vi "System_Configuration_Get.vi"(3 "error in (no error)":errorcluster, 4 "Device Selection":T1, 5 "Devices":T2) -> (0 "error out":errorcluster, 2 "Config":T3 {"Compute Config"."Post-Trigger Time" format="%.3f ms"; "Compute Config"."Pre-Trigger Time" format="%.3f ms"; "Compute Config"."Trigger Frequency" items=["Single", "Continuous"]; "Compute Config"."Trigger Type" items=["GPS Time", "Anomaly Detection"]; "SDR Config"."WRx 2\nGain Attenuation" min=0 max=27 step=1 scale=0.0..27.0; "SDR Config"."WRx 2\nRSSI Threshold" format="%.2f dBm"; "SDR Config"."WRx 2\nGain Mode" items=["Automatic", "Fixed"]; "SDR Config"."WRx 2\nBandwidth Mode" items=["500 MHz"]; "SDR Config"."WRx 2\nIF Frequency" items=["1200 MHz", "1400 MHz", "3000 MHZ"]; "SDR Config"."WRx 1\nGain Attenuation" min=0 max=27 step=1 scale=0.0..27.0; "SDR Config"."WRx 1\nRSSI Threshold" format="%.2f dBm"; "SDR Config"."WRx 1\nGain Mode" items=["Automatic", "Fixed"]; "SDR Config"."WRx 1\nBandwidth Mode" items=["500 MHz"]; "SDR Config"."WRx 1\nIF Frequency" items=["1200 MHz", "1400 MHz", "3000 MHZ"]})   [LabVIEW 2024]
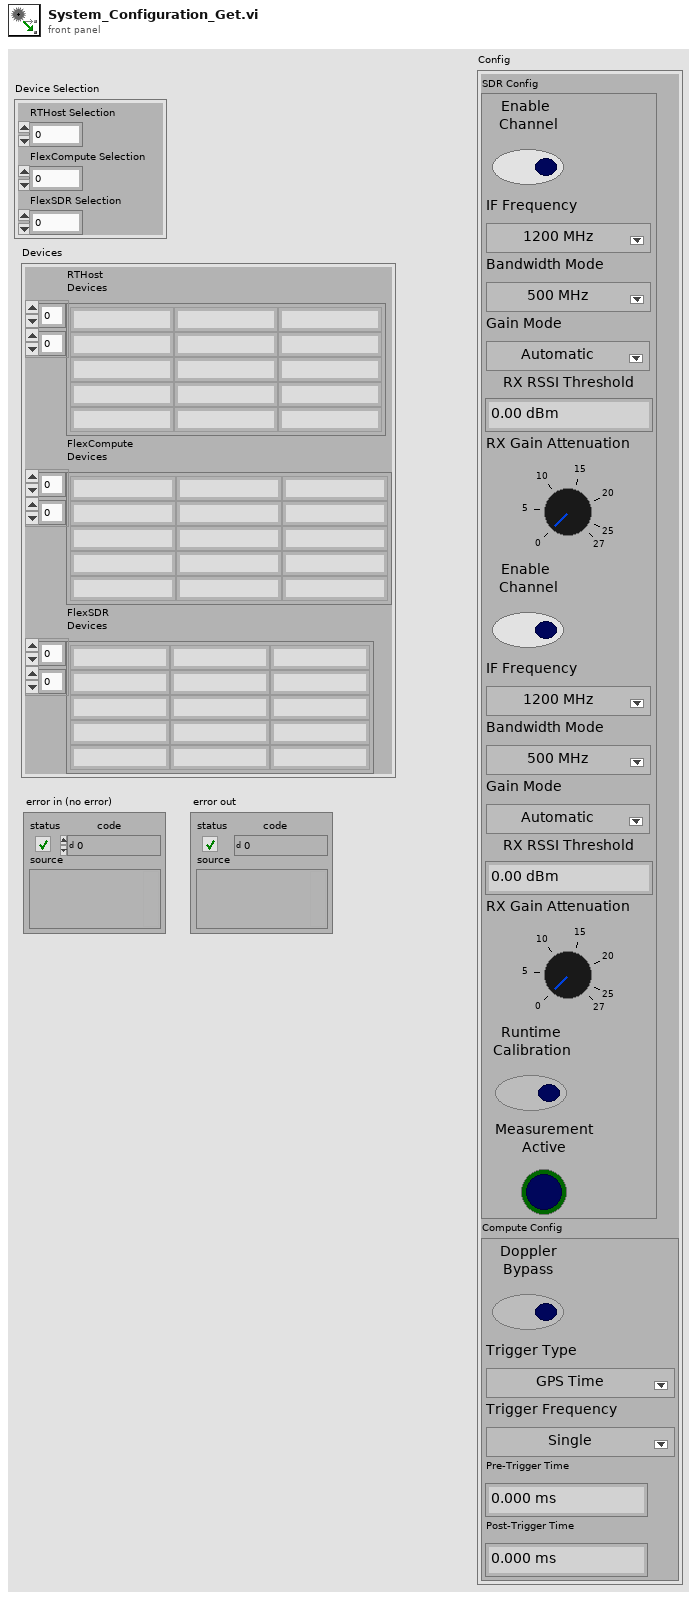
[diagram p1: front panel]
types:
  T1 = cluster{"RTHost Selection":u16, "FlexCompute Selection":u16, "FlexSDR Selection":u16}
  T2 = cluster{"RTHost\nDevices":string[][], "FlexCompute\nDevices":string[][], "FlexSDR\nDevices":string[][]}
  T3 = cluster{"SDR Config":cluster{"WRx 1\nEnable Channel":bool, "WRx 1\nIF Frequency":u16, "WRx 1\nBandwidth Mode":u16, "WRx 1\nGain Mode":u16, "WRx 1\nRSSI Threshold":dbl, "WRx 1\nGain Attenuation":i64, "WRx 2\nEnable Channel":bool, "WRx 2\nIF Frequency":u16, "WRx 2\nBandwidth Mode":u16, "WRx 2\nGain Mode":u16, "WRx 2\nRSSI Threshold":dbl, "WRx 2\nGain Attenuation":i64, "Runtime\nCalibration":bool, "Measurement\nActive":bool}, "Compute Config":cluster{"Doppler\nBypass":bool, "Trigger Type":u16, "Trigger Frequency":u16, "Pre-Trigger Time":dbl, "Post-Trigger Time":dbl}}
  T4 = cluster{"Doppler\nBypass":bool, "Trigger Type":u16, "Trigger Frequency":u16, "Pre-Trigger Time":dbl, "Post-Trigger Time":dbl}
  T5 = cluster{"WRx 1\nEnable Channel":bool, "WRx 1\nIF Frequency":u16, "WRx 1\nBandwidth Mode":u16, "WRx 1\nGain Mode":u16, "WRx 1\nRSSI Threshold":dbl, "WRx 1\nGain Attenuation":i64, "WRx 2\nEnable Channel":bool, "WRx 2\nIF Frequency":u16, "WRx 2\nBandwidth Mode":u16, "WRx 2\nGain Mode":u16, "WRx 2\nRSSI Threshold":dbl, "WRx 2\nGain Attenuation":i64, "Runtime\nCalibration":bool, "Measurement\nActive":bool}
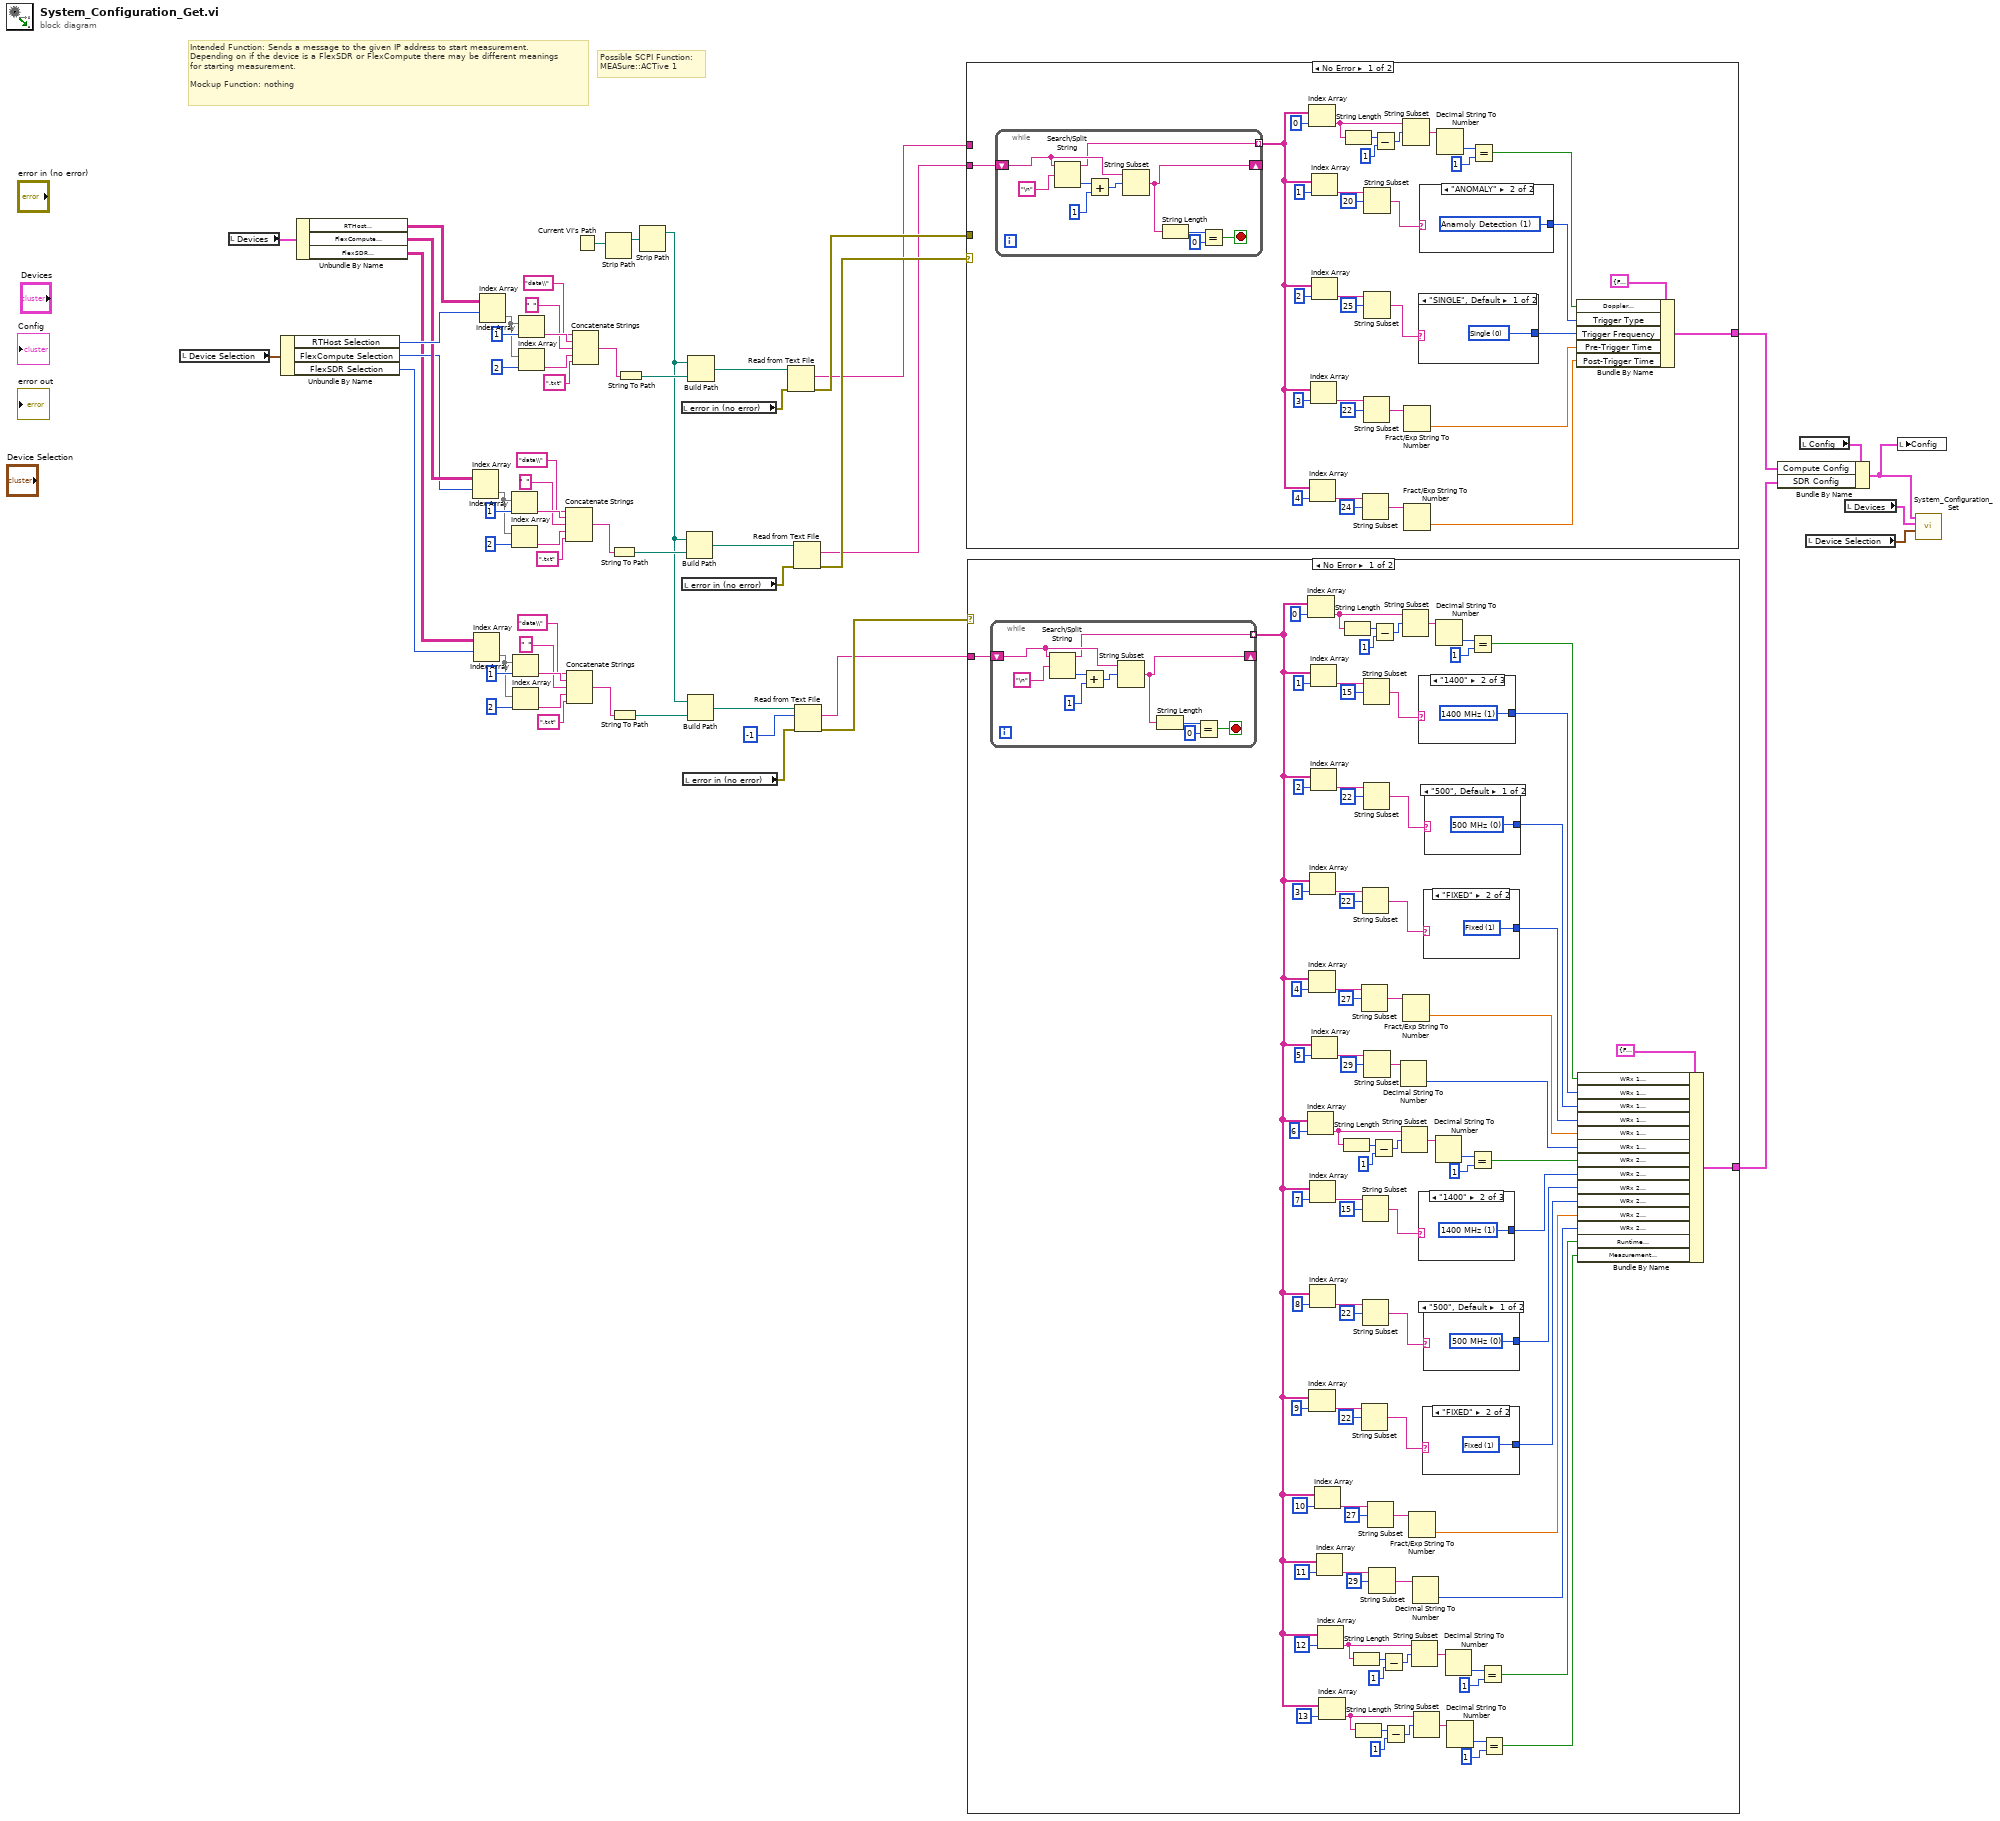
[diagram p0: block diagram]
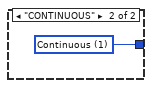
[diagram p2: hidden frame]
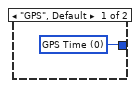
[diagram p3: hidden frame]
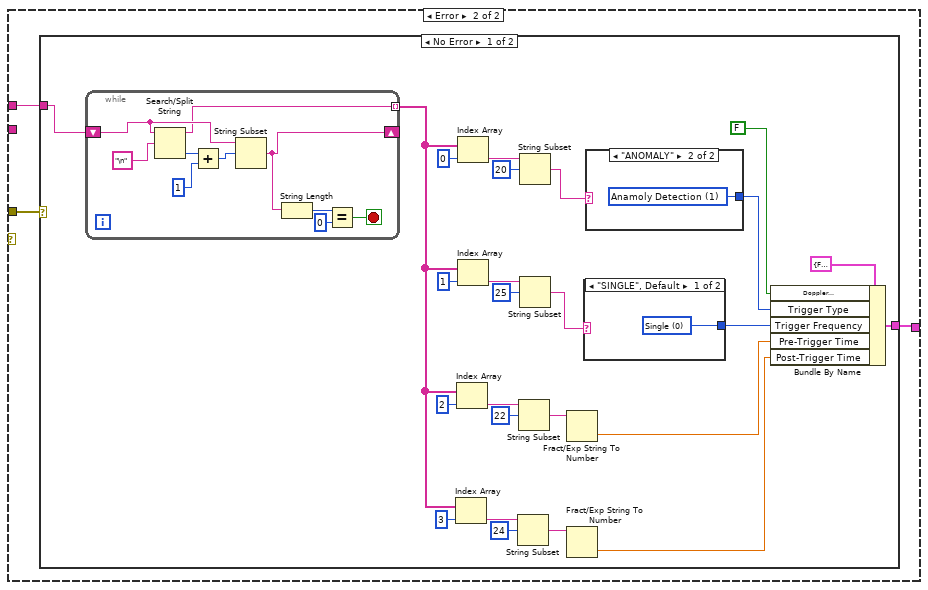
[diagram p4: hidden frame]
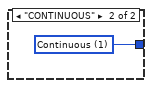
[diagram p5: hidden frame]
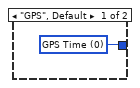
[diagram p6: hidden frame]
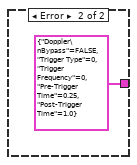
[diagram p7: hidden frame]
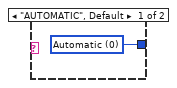
[diagram p8: hidden frame]
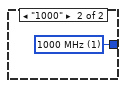
[diagram p9: hidden frame]
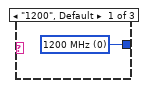
[diagram p10: hidden frame]
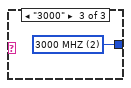
[diagram p11: hidden frame]
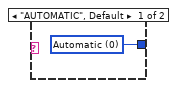
[diagram p12: hidden frame]
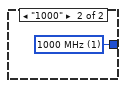
[diagram p13: hidden frame]
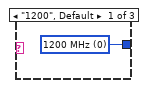
[diagram p14: hidden frame]
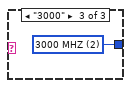
[diagram p15: hidden frame]
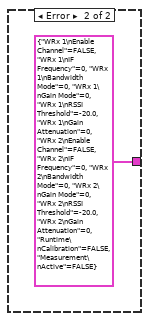
[diagram p16: hidden frame]
diagram:
  # "Possible SCPI Function:\nMEASure::ACTive 1"
  # "Intended Function: Sends a message to the given IP address to start measurement.\nDepending on if the device is a FlexSDR or FlexCompute there may be different meanings\nfor starting measurement.\n\nMockup Function: nothing"
  n1 = local read "Device Selection"() -> (w45:T1)
  n2 = local read "Devices"() -> (w49:T2)
  n3 = Unbundle By Name(w45) -> ("RTHost Selection"=w43:u16, "FlexCompute Selection"=w17:u16, "FlexSDR Selection"=w15:u16)
  n4 = Unbundle By Name(w49) -> ("RTHost\nDevices"=w44:string[][], "FlexCompute\nDevices"=w18:string[][], "FlexSDR\nDevices"=w16:string[][])
  n5 = Index Array(array=w18, index (row)=w17) -> (element=w41:string[])  [unwired: 1 in]
  n6 = Index Array(array=w16, index (row)=w15) -> (element=w29:string[])  [unwired: 1 in]
  n7 = Index Array(array=w44, index (row)=w43) -> (element=w58:string[])  [unwired: 1 in]
  n8 = Index Array(array=w41, index=1) -> (element=w39:string)
  n9 = Index Array(array=w41, index=2) -> (element=w38:string)
  n10 = Index Array(array=w29, index=1) -> (element=w27:string)
  n11 = Index Array(array=w29, index=2) -> (element=w26:string)
  n12 = Index Array(array=w58, index=1) -> (element=w56:string)
  n13 = Index Array(array=w58, index=2) -> (element=w55:string)
  n14 = Concatenate Strings("data\\" ("string"), w39, " " ("element"), w38, ".txt" ("string")) -> (w34:string)
  n15 = Concatenate Strings("data\\" ("string"), w27, " " ("element"), w26, ".txt" ("string")) -> (w22:string)
  n16 = Concatenate Strings("data\\" ("string"), w56, " " ("element"), w55, ".txt" ("string")) -> (w51:string)
  n17 = Current VI's Path() -> (path=w60:path)
  n18 = Strip Path(path=w60) -> (stripped path=w46:path)  [unwired: 1 out]
  n19 = String To Path(string=w34) -> (path=w33:path)
  n20 = String To Path(string=w22) -> (path=w21:path)
  n21 = String To Path(string=w51) -> (path=w50:path)
  n22 = Strip Path(path=w46) -> (stripped path=w19:path)  [unwired: 1 out]
  n23 = local read "error in (no error)"() -> (w48:errorcluster)
  n24 = local read "error in (no error)"() -> (w32:errorcluster)
  n25 = local read "error in (no error)"() -> (w20:errorcluster)
  n26 = Build Path(base path=w19, name or relative path=w33) -> (appended path=w31:path)
  n27 = Build Path(base path=w19, name or relative path=w21) -> (appended path=w11:path)
  n28 = Build Path(base path=w19, name or relative path=w50) -> (appended path=w47:path)
  n29 = Read from Text File(file (use dialog)=w47, error in=w48) -> (text=w7:string, error out=w14:errorcluster)  [unwired: 2 in, 2 out]
  n30 = Read from Text File(file (use dialog)=w31, error in=w32) -> (text=w8:string, error out=w13:errorcluster)  [unwired: 2 in, 2 out]
  n31 = Read from Text File(file (use dialog)=w11, count=-1, error in=w20) -> (text=w10:string, error out=w12:errorcluster)  [unwired: 1 in, 2 out]
  n32 = case shown="No Error" w13 {
    tunnel: w8 -> [w69 _]
    tunnel: w7 -> [_ w108]
    tunnel: w14 -> [_ w110]
    tunnel: [w61 w109] -> w5
    frame No Error {
      n33 = while {
        shift-right: [w99] -> _
        shift-left: w69 -> [w106]
        tunnel: [w98] -> w70 mode=indexing
        stop <- w100 stop-if-true
        n34 = Search/Split String(string=w106, search string/char (-)="\n") -> (substring before match=w98:string, offset of match=w105:i32)  [unwired: 1 in, 1 out]
        n35 = Add(x=w105, y=1) -> (x+y=w103:i32)
        n36 = String Subset(string=w106, offset (0)=w103) -> (substring=w99:string)  [unwired: 1 in]
        n37 = String Length(string=w99) -> (length=w102:i32)
        n38 = Equal?(x=w102, y=0) -> (x = y?=w100:bool)
      }
      n39 = Index Array(array=w70, index=0) -> (element=w90:string)
      n40 = Index Array(array=w70, index=4) -> (element=w73:string)
      n41 = Index Array(array=w70, index=3) -> (element=w76:string)
      n42 = Index Array(array=w70, index=1) -> (element=w84:string)
      n43 = Index Array(array=w70, index=2) -> (element=w80:string)
      n44 = String Length(string=w90) -> (length=w92:i32)
      n45 = String Subset(string=w73, offset (0)=24) -> (substring=w71:string)  [unwired: 1 in]
      n46 = String Subset(string=w76, offset (0)=22) -> (substring=w68:string)  [unwired: 1 in]
      n47 = String Subset(string=w84, offset (0)=20) -> (substring=w82:string)  [unwired: 1 in]
      n48 = String Subset(string=w80, offset (0)=25) -> (substring=w78:string)  [unwired: 1 in]
      n49 = Subtract(x=w92, y=1) -> (x-y=w89:i32)
      n50 = String Subset(string=w90, offset (0)=w89) -> (substring=w88:string)  [unwired: 1 in]
      n51 = Fract/Exp String To Number(string=w68) -> (number=w62:dbl)  [unwired: 3 in, 1 out]
      n52 = Fract/Exp String To Number(string=w71) -> (number=w63:dbl)  [unwired: 3 in, 1 out]
      n53 = case shown="\"SINGLE\", Default" w78 {
        tunnel: [w94 w95] -> w64
        frame "SINGLE", Default {
          w94 = u16 0 items=["Single", "Continuous"] ("Trigger Frequency")
        }
        frame "CONTINUOUS" {
          w95 = u16 1 items=["Single", "Continuous"] ("Trigger Frequency")
        }
      }
      n54 = case shown="\"ANOMALY\"" w82 {
        tunnel: [w96 w97] -> w65
        frame "GPS", Default {
          w96 = u16 0 items=["GPS Time", "Anamoly Detection"] ("Trigger Type")
        }
        frame "ANOMALY" {
          w97 = u16 1 items=["GPS Time", "Anamoly Detection"] ("Trigger Type")
        }
      }
      n55 = Decimal String To Number(string=w88) -> (number=w87:i32)  [unwired: 2 in, 1 out]
      n56 = Equal?(x=w87, y=1) -> (x = y?=w66:bool)
      n57 = Bundle By Name(cluster=T4 {"Doppler\nBypass"=FALSE, "Trigger Type"=0, "Trigger Frequency"=0, "Pre-Trigger Time"=0.25, "Post-Trigger Time"=1.0} ("Compute Config"), "Doppler\nBypass"=w66, "Trigger Type"=w65, "Trigger Frequency"=w64, "Pre-Trigger Time"=w62, "Post-Trigger Time"=w63) -> (w61:T4)
    }
    frame Error {
      n58 = case shown="No Error" w110 {
        tunnel: [w111 T4 {"Doppler\nBypass"=FALSE, "Trigger Type"=0, "Trigger Frequency"=0, "Pre-Trigger Time"=0.25, "Post-Trigger Time"=1.0} ("Compute Config")] -> w109
        tunnel: w108 -> [w113 _]
        frame No Error {
          n59 = while {
            shift-right: [w141] -> _
            shift-left: w113 -> [w148]
            tunnel: [w140] -> w120 mode=indexing
            stop <- w142 stop-if-true
            n60 = Search/Split String(string=w148, search string/char (-)="\n") -> (substring before match=w140:string, offset of match=w147:i32)  [unwired: 1 in, 1 out]
            n61 = Add(x=w147, y=1) -> (x+y=w145:i32)
            n62 = String Subset(string=w148, offset (0)=w145) -> (substring=w141:string)  [unwired: 1 in]
            n63 = String Length(string=w141) -> (length=w144:i32)
            n64 = Equal?(x=w144, y=0) -> (x = y?=w142:bool)
          }
          n65 = Index Array(array=w120, index=3) -> (element=w123:string)
          n66 = Index Array(array=w120, index=2) -> (element=w126:string)
          n67 = Index Array(array=w120, index=0) -> (element=w134:string)
          n68 = Index Array(array=w120, index=1) -> (element=w130:string)
          n69 = String Subset(string=w123, offset (0)=24) -> (substring=w121:string)  [unwired: 1 in]
          n70 = String Subset(string=w126, offset (0)=22) -> (substring=w119:string)  [unwired: 1 in]
          n71 = String Subset(string=w134, offset (0)=20) -> (substring=w132:string)  [unwired: 1 in]
          n72 = String Subset(string=w130, offset (0)=25) -> (substring=w128:string)  [unwired: 1 in]
          n73 = Fract/Exp String To Number(string=w119) -> (number=w114:dbl)  [unwired: 3 in, 1 out]
          n74 = Fract/Exp String To Number(string=w121) -> (number=w115:dbl)  [unwired: 3 in, 1 out]
          n75 = case shown="\"SINGLE\", Default" w128 {
            tunnel: [w136 w137] -> w116
            frame "SINGLE", Default {
              w136 = u16 0 items=["Single", "Continuous"] ("Trigger Frequency")
            }
            frame "CONTINUOUS" {
              w137 = u16 1 items=["Single", "Continuous"] ("Trigger Frequency")
            }
          }
          n76 = case shown="\"ANOMALY\"" w132 {
            tunnel: [w138 w139] -> w117
            frame "GPS", Default {
              w138 = u16 0 items=["GPS Time", "Anamoly Detection"] ("Trigger Type")
            }
            frame "ANOMALY" {
              w139 = u16 1 items=["GPS Time", "Anamoly Detection"] ("Trigger Type")
            }
          }
          n77 = Bundle By Name(cluster=T4 {"Doppler\nBypass"=FALSE, "Trigger Type"=0, "Trigger Frequency"=0, "Pre-Trigger Time"=0.25, "Post-Trigger Time"=1.0} ("Compute Config"), "Doppler\nBypass"=FALSE ("Doppler\nBypass"), "Trigger Type"=w117, "Trigger Frequency"=w116, "Pre-Trigger Time"=w114, "Post-Trigger Time"=w115) -> (w111:T4)
        }
        frame Error {
        }
      }
    }
  }
  n78 = case shown="No Error" w12 {
    tunnel: w10 -> [w240 _]
    tunnel: [w151 T5 {"WRx 1\nEnable Channel"=FALSE, "WRx 1\nIF Frequency"=0, "WRx 1\nBandwidth Mode"=0, "WRx 1\nGain Mode"=0, "WRx 1\nRSSI Threshold"=-20.0, "WRx 1\nGain Attenuation"=0, "WRx 2\nEnable Channel"=FALSE, "WRx 2\nIF Frequency"=0, "WRx 2\nBandwidth Mode"=0, "WRx 2\nGain Mode"=0, "WRx 2\nRSSI Threshold"=-20.0, "WRx 2\nGain Attenuation"=0, "Runtime\nCalibration"=FALSE, "Measurement\nActive"=FALSE} ("SDR Config")] -> w4
    frame No Error {
      n79 = while {
        shift-right: [w256] -> _
        shift-left: w240 -> [w263]
        tunnel: [w255] -> w169 mode=indexing
        stop <- w257 stop-if-true
        n80 = Search/Split String(string=w263, search string/char (-)="\n") -> (substring before match=w255:string, offset of match=w262:i32)  [unwired: 1 in, 1 out]
        n81 = Add(x=w262, y=1) -> (x+y=w260:i32)
        n82 = String Subset(string=w263, offset (0)=w260) -> (substring=w256:string)  [unwired: 1 in]
        n83 = String Length(string=w256) -> (length=w259:i32)
        n84 = Equal?(x=w259, y=0) -> (x = y?=w257:bool)
      }
      n85 = Index Array(array=w169, index=6) -> (element=w209:string)
      n86 = Index Array(array=w169, index=0) -> (element=w236:string)
      n87 = Index Array(array=w169, index=4) -> (element=w218:string)
      n88 = Index Array(array=w169, index=9) -> (element=w195:string)
      n89 = Index Array(array=w169, index=3) -> (element=w222:string)
      n90 = Index Array(array=w169, index=7) -> (element=w203:string)
      n91 = Index Array(array=w169, index=8) -> (element=w199:string)
      n92 = Index Array(array=w169, index=1) -> (element=w230:string)
      n93 = Index Array(array=w169, index=2) -> (element=w226:string)
      n94 = Index Array(array=w169, index=5) -> (element=w214:string)
      n95 = Index Array(array=w169, index=10) -> (element=w191:string)
      n96 = Index Array(array=w169, index=11) -> (element=w187:string)
      n97 = Index Array(array=w169, index=12) -> (element=w182:string)
      n98 = Index Array(array=w169, index=13) -> (element=w174:string)
      n99 = String Length(string=w209) -> (length=w211:i32)
      n100 = String Length(string=w236) -> (length=w238:i32)
      n101 = String Length(string=w182) -> (length=w184:i32)
      n102 = String Length(string=w174) -> (length=w176:i32)
      n103 = String Subset(string=w218, offset (0)=27) -> (substring=w216:string)  [unwired: 1 in]
      n104 = String Subset(string=w195, offset (0)=22) -> (substring=w193:string)  [unwired: 1 in]
      n105 = String Subset(string=w222, offset (0)=22) -> (substring=w220:string)  [unwired: 1 in]
      n106 = String Subset(string=w203, offset (0)=15) -> (substring=w201:string)  [unwired: 1 in]
      n107 = String Subset(string=w199, offset (0)=22) -> (substring=w197:string)  [unwired: 1 in]
      n108 = String Subset(string=w230, offset (0)=15) -> (substring=w228:string)  [unwired: 1 in]
      n109 = String Subset(string=w226, offset (0)=22) -> (substring=w224:string)  [unwired: 1 in]
      n110 = String Subset(string=w214, offset (0)=29) -> (substring=w162:string)  [unwired: 1 in]
      n111 = String Subset(string=w191, offset (0)=27) -> (substring=w189:string)  [unwired: 1 in]
      n112 = String Subset(string=w187, offset (0)=29) -> (substring=w157:string)  [unwired: 1 in]
      n113 = Subtract(x=w211, y=1) -> (x-y=w208:i32)
      n114 = Subtract(x=w238, y=1) -> (x-y=w235:i32)
      n115 = Subtract(x=w184, y=1) -> (x-y=w181:i32)
      n116 = Subtract(x=w176, y=1) -> (x-y=w173:i32)
      n117 = Decimal String To Number(string=w162) -> (number=w161:i32)  [unwired: 2 in, 1 out]
      n118 = String Subset(string=w209, offset (0)=w208) -> (substring=w207:string)  [unwired: 1 in]
      n119 = String Subset(string=w236, offset (0)=w235) -> (substring=w234:string)  [unwired: 1 in]
      n120 = Fract/Exp String To Number(string=w216) -> (number=w163:dbl)  [unwired: 3 in, 1 out]
      n121 = Fract/Exp String To Number(string=w189) -> (number=w155:dbl)  [unwired: 3 in, 1 out]
      n122 = String Subset(string=w182, offset (0)=w181) -> (substring=w180:string)  [unwired: 1 in]
      n123 = Decimal String To Number(string=w157) -> (number=w156:i32)  [unwired: 2 in, 1 out]
      n124 = String Subset(string=w174, offset (0)=w173) -> (substring=w172:string)  [unwired: 1 in]
      n125 = case shown="\"1400\"" w201 {
        tunnel: [w245 w246 w247] -> w152
        frame "1200", Default {
          w245 = u16 0 items=["1200 MHz", "1400 MHz", "3000 MHZ"] ("WRx 1\nIF Frequency")
        }
        frame "1400" {
          w246 = u16 1 items=["1200 MHz", "1400 MHz", "3000 MHZ"] ("WRx 1\nIF Frequency")
        }
        frame "3000" {
          w247 = u16 2 items=["1200 MHz", "1400 MHz", "3000 MHZ"] ("WRx 1\nIF Frequency")
        }
      }
      n126 = case shown="\"1400\"" w228 {
        tunnel: [w252 w253 w254] -> w166
        frame "1200", Default {
          w252 = u16 0 items=["1200 MHz", "1400 MHz", "3000 MHZ"] ("WRx 1\nIF Frequency")
        }
        frame "1400" {
          w253 = u16 1 items=["1200 MHz", "1400 MHz", "3000 MHZ"] ("WRx 1\nIF Frequency")
        }
        frame "3000" {
          w254 = u16 2 items=["1200 MHz", "1400 MHz", "3000 MHZ"] ("WRx 1\nIF Frequency")
        }
      }
      n127 = case shown="\"FIXED\"" w193 {
        tunnel: [w241 w242] -> w154
        frame "AUTOMATIC", Default {
          w241 = u16 0 items=["Automatic", "Fixed"] ("WRx 1\nGain Mode")
        }
        frame "FIXED" {
          w242 = u16 1 items=["Automatic", "Fixed"] ("WRx 1\nGain Mode")
        }
      }
      n128 = case shown="\"FIXED\"" w220 {
        tunnel: [w248 w249] -> w164
        frame "AUTOMATIC", Default {
          w248 = u16 0 items=["Automatic", "Fixed"] ("WRx 1\nGain Mode")
        }
        frame "FIXED" {
          w249 = u16 1 items=["Automatic", "Fixed"] ("WRx 1\nGain Mode")
        }
      }
      n129 = case shown="\"500\", Default" w197 {
        tunnel: [w243 w244] -> w153
        frame "500", Default {
          w243 = u16 0 items=["500 MHz", "1000 MHz"] ("WRx 1\nBandwidth Mode")
        }
        frame "1000" {
          w244 = u16 1 items=["500 MHz", "1000 MHz"] ("WRx 1\nBandwidth Mode")
        }
      }
      n130 = case shown="\"500\", Default" w224 {
        tunnel: [w250 w251] -> w165
        frame "500", Default {
          w250 = u16 0 items=["500 MHz", "1000 MHz"] ("WRx 1\nBandwidth Mode")
        }
        frame "1000" {
          w251 = u16 1 items=["500 MHz", "1000 MHz"] ("WRx 1\nBandwidth Mode")
        }
      }
      n131 = Decimal String To Number(string=w207) -> (number=w206:i32)  [unwired: 2 in, 1 out]
      n132 = Decimal String To Number(string=w234) -> (number=w233:i32)  [unwired: 2 in, 1 out]
      n133 = Decimal String To Number(string=w180) -> (number=w179:i32)  [unwired: 2 in, 1 out]
      n134 = Decimal String To Number(string=w172) -> (number=w171:i32)  [unwired: 2 in, 1 out]
      n135 = Equal?(x=w206, y=1) -> (x = y?=w160:bool)
      n136 = Equal?(x=w233, y=1) -> (x = y?=w167:bool)
      n137 = Equal?(x=w179, y=1) -> (x = y?=w158:bool)
      n138 = Equal?(x=w171, y=1) -> (x = y?=w159:bool)
      n139 = Bundle By Name(cluster=T5 {"WRx 1\nEnable Channel"=FALSE, "WRx 1\nIF Frequency"=0, "WRx 1\nBandwidth Mode"=0, "WRx 1\nGain Mode"=0, "WRx 1\nRSSI Threshold"=-20.0, "WRx 1\nGain Attenuation"=0, "WRx 2\nEnable Channel"=FALSE, "WRx 2\nIF Frequency"=0, "WRx 2\nBandwidth Mode"=0, "WRx 2\nGain Mode"=0, "WRx 2\nRSSI Threshold"=-20.0, "WRx 2\nGain Attenuation"=0, "Runtime\nCalibration"=FALSE, "Measurement\nActive"=FALSE} ("SDR Config"), "WRx 1\nEnable Channel"=w167, "WRx 1\nIF Frequency"=w166, "WRx 1\nBandwidth Mode"=w165, "WRx 1\nGain Mode"=w164, "WRx 1\nRSSI Threshold"=w163, "WRx 1\nGain Attenuation"=w161, "WRx 2\nEnable Channel"=w160, "WRx 2\nIF Frequency"=w152, "WRx 2\nBandwidth Mode"=w153, "WRx 2\nGain Mode"=w154, "WRx 2\nRSSI Threshold"=w155, "WRx 2\nGain Attenuation"=w156, "Runtime\nCalibration"=w158, "Measurement\nActive"=w159) -> (w151:T5)
    }
    frame Error {
    }
  }
  n140 = local read "Config"() -> (w6:T3)
  n141 = Bundle By Name(cluster=w6, "Compute Config"=w5, "SDR Config"=w4) -> (w3:T3)
  n142 = local read "Device Selection"() -> (w1:T1)
  n143 = local read "Devices"() -> (w2:T2)
  n144 = local write "Config"(w3) -> ()
  n145 = call "System_Configuration_Set.vi"("Device Selection"=w1, "Devices"=w2, "Config"=w3) -> ()  [unwired: 4 in]
